vi "Update.vi"(8 "error in (no error)":errorcluster, 10 "Audio Data In":dbl[][](array[numeric]), 11 "Effect in":refnum<class "Effect.lvclass">) -> (0 "error out":errorcluster, 2 "Audio Data Out":dbl[][](array[numeric]), 3 "Effect out":refnum<class "Effect.lvclass">)   [LabVIEW 2018, in "Effect.lvclass"]
uses:
  Effect.lvclass
  Effect.lvclass/Effect.ctl
  Plugin Interfaces/Effect Interface/Effect Interface.lvlibp/Effect Interface Class/Effect Interface.lvclass
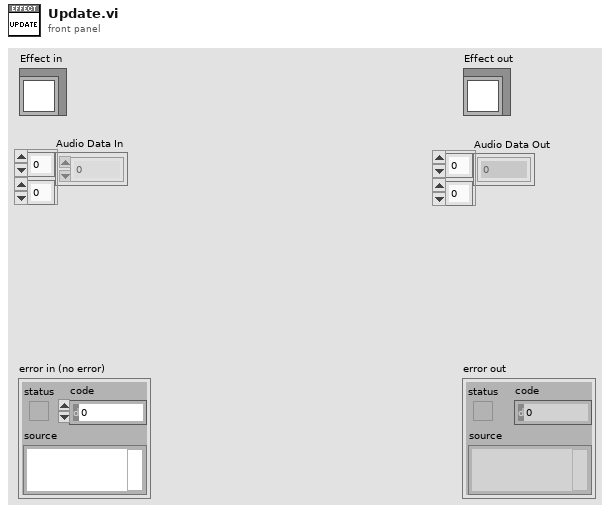
[diagram p1: front panel]
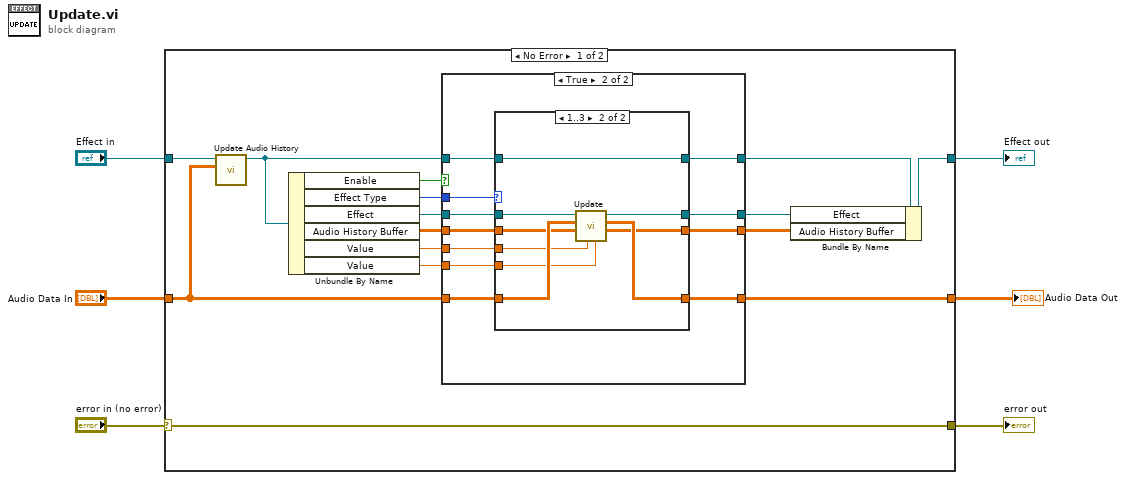
[diagram p0: block diagram]
diagram:
  n1 = case shown="No Error" "error in (no error)" {
    selector: "error in (no error)" -> [w21 w52]
    tunnel: [w21 w52] -> w5
    tunnel: [w9 w51] -> w3
    tunnel: "Effect in" -> [w20 w51]
    tunnel: "Audio Data In" -> [w18 w50]
    tunnel: [w19 w50] -> w1
    frame No Error {
      n2 = call "Update Audio History.vi"("Audio Data In"=w18, "Effect in"=w20) -> ("Effect out"=w15:refnum<class "Effect.lvclass">)  [unwired: 8 in, 1 out]
      n3 = Unbundle By Name(w15) -> ("Enable"=w17:bool, "Effect Type"=w16:i32, "Effect"=w14:refnum<class "Effect Interface.lvclass">, "Audio History Buffer"=w13:dbl[][], "Value"=w12:dbl, "Value"=w11:dbl)
      n4 = case shown="True" w17 {
        tunnel: [w25 w36] -> w19
        tunnel: w18 -> [w25 w35]
        tunnel: w16 -> [_ w34]
        tunnel: [w24 w33] -> w10
        tunnel: w15 -> [w24 w32]
        tunnel: w14 -> [w23 w31]
        tunnel: w13 -> [w22 w30]
        tunnel: w12 -> [_ w29]
        tunnel: w11 -> [_ w28]
        tunnel: [w23 w27] -> w8
        tunnel: [w22 w26] -> w7
        frame False {
        }
        frame True {
          n5 = case shown="1..3" w34 {
            tunnel: [w40 w47] -> w36
            tunnel: w35 -> [w40 w48]
            tunnel: [w39 w46] -> w33
            tunnel: w32 -> [w39 w46]
            tunnel: w31 -> [w38 w49]
            tunnel: w30 -> [w37 w45]
            tunnel: w29 -> [_ w44]
            tunnel: w28 -> [_ w43]
            tunnel: [w38 w42] -> w27
            tunnel: [w37 w41] -> w26
            frame Default {
            }
            frame 1..3 {
              n6 = call-dynamic "Update.vi"("Value2"=w43, "Value1"=w44, "Audio History Buffer In"=w45, "Audio Data In"=w48, "Effect Interface in"=w49) -> ("Audio History Buffer Out"=w41:dbl[][], "Audio Data Out"=w47:dbl[][], "Effect Interface out"=w42:refnum<class "Effect Interface.lvclass">)  [unwired: 3 in, 1 out]
            }
          }
        }
      }
      n7 = Bundle By Name(cluster=w10, "Effect"=w8, "Audio History Buffer"=w7) -> (w9:refnum<class "Effect.lvclass">)
    }
    frame Error {
    }
  }
  "error out" <- w5
  "Effect out" <- w3
  "Audio Data Out" <- w1
